vi "_FPGA_CycleAccumulator.vi"(1 "Init":bool, 2 "aux decycle in":u64) -> (5 "AuxCyc out":u64)   [LabVIEW 2018]
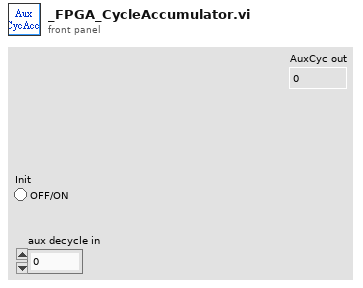
[diagram p1: front panel]
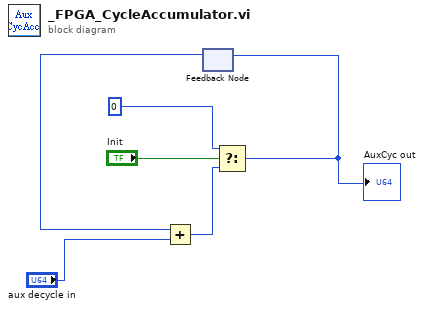
[diagram p0: block diagram]
diagram:
  n1 = feedback #1() -> (w1:u64)  [unwired: 1 in]
  n2 = Add(x=w1, y="aux decycle in") -> (x+y=w3:u64)
  n3 = Select(t=u64 0 ("aux decycle in 2"), s="Init", f=w3) -> (s? t:f=w2:u64)
  "AuxCyc out" <- w2
  n4 = feedback-in #1(w2) -> ()
